vi "发送指令-汇川机械手.vi"(1 "A":string="0", 2 "Y":string="0", 3 "X":string="0") -> (0 "发送指令":string)   [LabVIEW 2016]
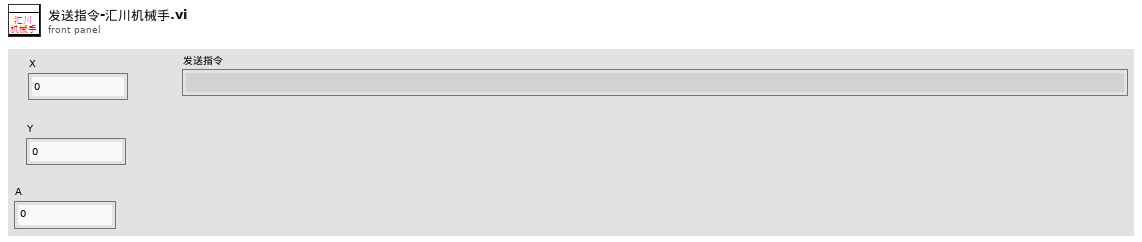
[diagram p1: front panel]
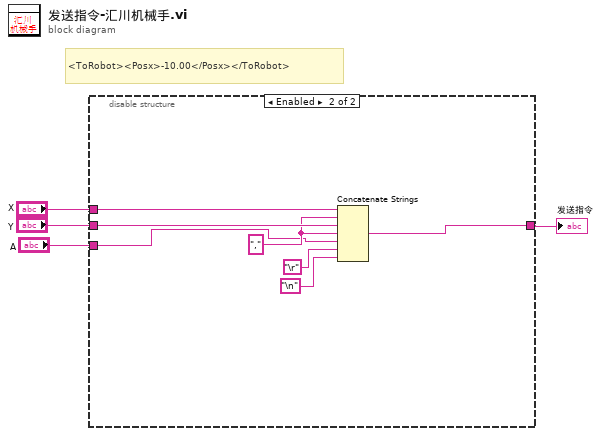
[diagram p0: block diagram]
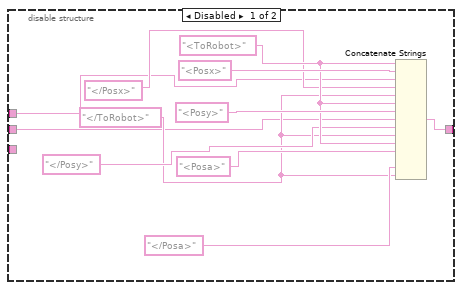
[diagram p2: hidden frame]
diagram:
  # "<ToRobot><Posx>-10.00</Posx></ToRobot>"
  n1 = disable-structure shown="Enabled" {
    disable-tunnel: [w16 w21] -> w4
    disable-tunnel: "X" -> [w7 w23]
    disable-tunnel: "Y" -> [w6 w22]
    disable-tunnel: "A" -> [_ w17]
    frame Disabled {
      w8 = "</ToRobot>"
      w12 = "<ToRobot>"
      n2 = Concatenate Strings(w12, "<Posx>", w7, "</Posx>", w8, w12, "<Posy>", w6, "</Posy>", w8, w12, "<Posa>", "</Posa>", w8) -> (w16:string, w5:string)
    }
    frame Enabled {
      w18 = "," ("字符串")
      n3 = Concatenate Strings(w23, w18, w22, w18, w17, "\r", "\n") -> (w21:string)
    }
  }
  "发送指令" <- w4
